vi "SetTrigger.vi"(8 "error in (no error)":errorcluster, 10 "Settings.Trigger":T1, 11 "Point Grey Camera in":refnum<class "Point Grey Camera.lvclass">) -> (0 "error out":errorcluster, 2 "Settings.Trigger  out":T1, 3 "Point Grey Camera out":refnum<class "Point Grey Camera.lvclass">)   [LabVIEW 2020, in "Point Grey Camera.lvclass"]
uses:
  Point Grey Camera.lvclass
  OnOffTypeDef.ctl
  Point Grey Camera.lvclass/Point Grey Camera.ctl
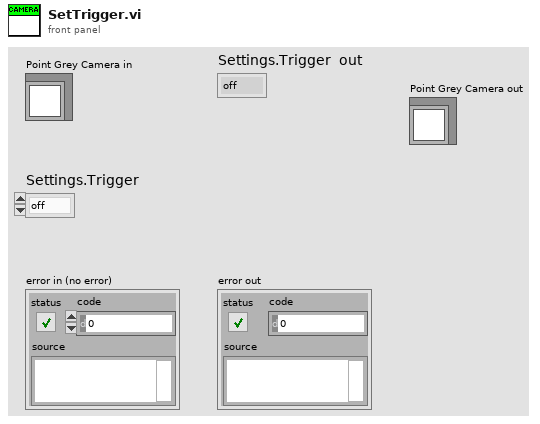
[diagram p1: front panel]
types:
  T1 = typedef "OnOffTypeDef.ctl" = enum16{"off", "on"}
  T2 = typedef "TriggerModeString_TypDEf.ctl" = cluster{"On":string, "Off":string}
  T3 = typedef "IMAQdx.ctl" = refnum<k21>
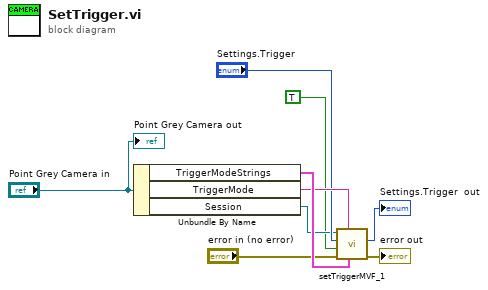
[diagram p0: block diagram]
diagram:
  n1 = Unbundle By Name("Point Grey Camera in") -> ("TriggerModeStrings"=w9:T2, "TriggerMode"=w8:string, "Session"=w4:T3)
  n2 = call "setTriggerMVF_1.vi"("TriggerModeStrings"=w9, "TrigerModeName"=w8, "error in"="error in (no error)", "cam connected"=TRUE, "Settings.Trigger"="Settings.Trigger", "Session"=w4) -> ("error out"=→"error out":errorcluster, "Settings.Trigger  out"=→"Settings.Trigger  out":T1)  [unwired: 2 in]
  "Point Grey Camera out" <- "Point Grey Camera in"
